vi "pop_boolean_array.vi"(8 "error in (no error)":errorcluster, 11 "Lua in":refnum<class "Lua.lvclass">) -> (0 "error out":errorcluster, 2 "value":bool[](array[boolean]), 3 "Lua out":refnum<class "Lua.lvclass">)   [LabVIEW 2020, in "Lua for LabVIEW.lvlib" / "Lua.lvclass"]
doc: "Pop a numeric value from the stack."
uses:
  Lua.lvclass
  Lua.lvclass/Lua.ctl
  lib/lua.dll/types/lua_error_code_offset.vi
  lib/lua.dll/lua_settop.vi
  <vilib>/Utility/error.llb/Error Cluster From Error Code.vi
  lib/lua.dll/lua.dll.lvlib
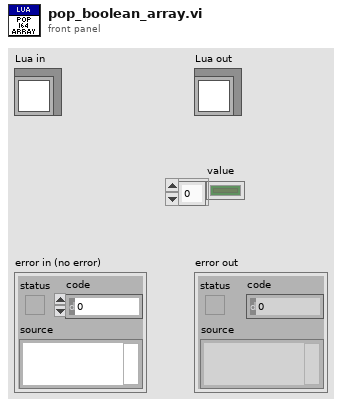
[diagram p1: front panel]
types:
  T1 = typedef "lua.dll.lvlib/lua_types.ctl" = i32
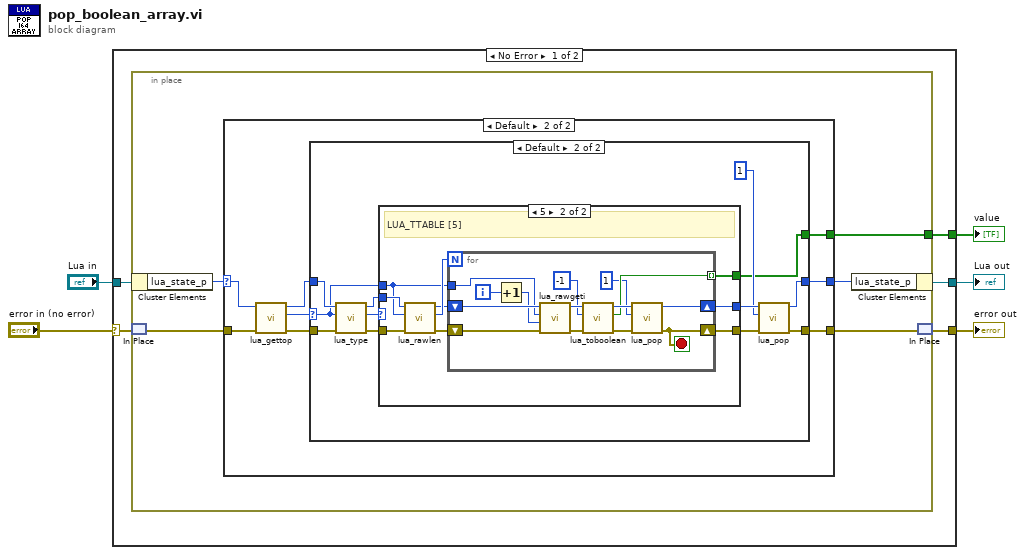
[diagram p0: block diagram]
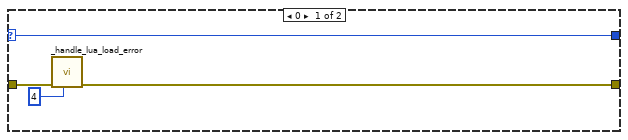
[diagram p2: hidden frame]
diagram:
  n1 = case shown="No Error" "error in (no error)" {
    selector: "error in (no error)" -> [w7 w68]
    tunnel: [w8 w68] -> w2
    tunnel: [w9 w67] -> w3
    tunnel: "Lua in" -> [w10 w67]
    tunnel: [w6 _] -> w1
    frame No Error {
      n2 = in-place {
        in-place-border: [w11] -> w6
        n3 = in-place-cluster #1(w10) -> ("lua_state_p"=w14:u64)
        n4 = in-place-match #2(w7) -> (w13:errorcluster)
        n5 = case shown="Default" w14 {
          selector: w14 -> [w19 w23]
          tunnel: [w19 w27] -> w15
          tunnel: w13 -> [w16 w24]
          tunnel: [w17 w26] -> w12
          tunnel: [_ w25] -> w11
          frame 0 {
            n6 = call "_handle_lua_load_error.vi"("lua_load errcode"=4, "error in (no error)"=w16) -> ("error out"=w17:errorcluster)  [unwired: 9 in]
          }
          frame Default {
            n7 = call "lua_gettop.vi"("error in (no error)"=w24, "lua_state_p"=w23) -> ("error out"=w21:errorcluster, "index"=w20:i32, "lua_state_p out"=w22:u64)  [unwired: 7 in]
            n8 = case shown="Default" w20 {
              selector: w20 -> [_ w30]
              tunnel: [w28 w38] -> w27
              tunnel: [w29 w37] -> w26
              tunnel: [_ w33] -> w25
              tunnel: w22 -> [w28 w32]
              tunnel: w21 -> [w29 w31]
              frame 0 {
              }
              frame Default {
                n9 = call "lua_type.vi"("error in (no error)"=w31, "index"=w30, "lua_state_p"=w32) -> ("error out"=w34:errorcluster, "lua type"=w41:T1, "lua_state_p out"=w40:u64)  [unwired: 6 in]
                n10 = case shown="5" w41 {
                  tunnel: [w42 w45] -> w39
                  tunnel: w40 -> [w42 w52]
                  tunnel: [w43 w46] -> w35
                  tunnel: w34 -> [w43 w51]
                  tunnel: [_ w47] -> w33
                  tunnel: w30 -> [_ w44]
                  frame Default {
                  }
                  frame 5 {
                    # "LUA_TTABLE [5]"
                    n11 = call "lua_rawlen.vi"("error in (no error)"=w51, "index"=w44, "lua_state_p"=w52) -> ("error out"=w48:errorcluster, "length"=w50:u64, "lua_state_p out"=w49:u64)  [unwired: 6 in]
                    n12 = for {
                      N: w50 -> [_]
                      shift-right: [w57] -> w45
                      shift-left: w49 -> [w66]
                      shift-right: [w54] -> w46
                      shift-left: w48 -> [w61]
                      tunnel: [w58] -> w47 mode=indexing
                      tunnel: w44 -> [w53]
                      i -> [w65]
                      stop <- w54 stop-if-true
                      n13 = Increment(x=w65) -> (x+1=w64:i32)
                      n14 = call "lua_rawgeti.vi"("error in (no error)"=w61, "n"=w64, "index"=w53, "lua_state_p"=w66) -> ("error out"=w62:errorcluster, "lua_state_p out"=w63:u64)  [unwired: 5 in, 1 out]
                      n15 = call "lua_toboolean.vi"("error in (no error)"=w62, "index"=-1, "lua_state_p"=w63) -> ("error out"=w55:errorcluster, "boolean"=w58:bool, "lua_state_p out"=w59:u64)  [unwired: 6 in]
                      n16 = call "lua_pop.vi"("error in (no error)"=w55, "n"=1, "lua_state_p"=w59) -> ("error out"=w54:errorcluster, "lua_state_p out"=w57:u64)  [unwired: 7 in]
                    }
                  }
                }
                n17 = call "lua_pop.vi"("error in (no error)"=w35, "n"=1, "lua_state_p"=w39) -> ("error out"=w37:errorcluster, "lua_state_p out"=w38:u64)  [unwired: 7 in]
              }
            }
          }
        }
        n18 = in-place-cluster #1("lua_state_p"=w15) -> (w9:refnum<class "Lua.lvclass">)
        n19 = in-place-match #2(w12) -> (w8:errorcluster)
      }
    }
    frame Error {
    }
  }
  "error out" <- w2
  "Lua out" <- w3
  "value" <- w1
